vi "drive_getInputs.vi"(11 "Joysticks":T2) -> (3 "Drive":T1)   [LabVIEW 2013]
uses:
  util/joystick_vals.ctl
  <vilib>/Rock Robotics/WPI/Joystick/WPI_JoystickButtonState.ctl
  drive_inputs.ctl
panel:
  out "Angular Rate":dbl
  in  "Drive 2":T1
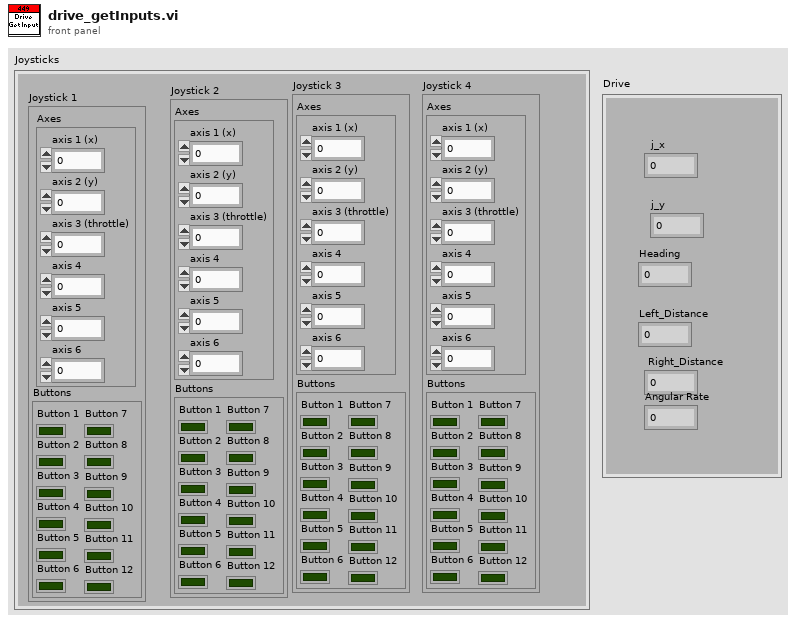
[diagram p1: front panel]
types:
  T1 = typedef "drive_inputs.ctl" = cluster{"j_x":dbl, "j_y":dbl, "Heading":dbl, "Left_Distance":dbl, " Right_Distance":dbl}
  T2 = typedef "joystick_vals.ctl" = cluster{"Joystick 1":cluster{"Axes":cluster{"axis 1 (x)":dbl, "axis 2 (y)":dbl, "axis 3 (throttle)":dbl, "axis 4":dbl, "axis 5":dbl, "axis 6":dbl}, "Buttons":T3}, "Joystick 2":cluster{"Axes":cluster{"axis 1 (x)":dbl, "axis 2 (y)":dbl, "axis 3 (throttle)":dbl, "axis 4":dbl, "axis 5":dbl, "axis 6":dbl}, "Buttons":T3}, "Joystick 3":cluster{"Axes":cluster{"axis 1 (x)":dbl, "axis 2 (y)":dbl, "axis 3 (throttle)":dbl, "axis 4":dbl, "axis 5":dbl, "axis 6":dbl}, "Buttons":T3}, "Joystick 4":cluster{"Axes":cluster{"axis 1 (x)":dbl, "axis 2 (y)":dbl, "axis 3 (throttle)":dbl, "axis 4":dbl, "axis 5":dbl, "axis 6":dbl}, "Buttons":T3}}
  T3 = typedef "WPI_JoystickButtonState.ctl" = cluster{"Button 1":bool, "Button 2":bool, "Button 3":bool, "Button 4":bool, "Button 5":bool, "Button 6":bool, "Button 7":bool, "Button 8":bool, "Button 9":bool, "Button 10":bool, "Button 11":bool, "Button 12":bool}
  T4 = cluster{"Axes":cluster{"axis 1 (x)":dbl, "axis 2 (y)":dbl, "axis 3 (throttle)":dbl, "axis 4":dbl, "axis 5":dbl, "axis 6":dbl}, "Buttons":T3}
  T5 = cluster{"axis 1 (x)":dbl, "axis 2 (y)":dbl, "axis 3 (throttle)":dbl, "axis 4":dbl, "axis 5":dbl, "axis 6":dbl}
  T6 = typedef "WPI_EncoderDevRef.ctl" = cluster{"DevStatus":errorcluster, "EncoderIndex":T7, "CounterIndex":T8, "DistancePerCount":dbl, "Decoding Type":T9}
  T7 = typedef "FPGA_EncoderIdx.ctl" = enum8{"Enc 0", "Enc 1", "Enc 2", "Enc 3", "Invalid"}
  T8 = typedef "FPGA_CounterCtrSystemIndex.ctl" = enum8{"Ctr 0", "Ctr 1", "Ctr 2", "Ctr 3", "Ctr 4", "Ctr 5", "Ctr 6", "Ctr 7", "Invalid"}
  T9 = typedef "WPI_EncoderType.ctl" = enum16{"1x", "2x", "4x"}
  T10 = typedef "WPI_GyroDevRef.ctl" = cluster{"DevStatus":errorcluster, "Analog Module":T11, "Analog Channel":T12, "Offset":dbl, "Gain (VoltsPerDegree/Second)":dbl}
  T11 = typedef "FPGA_TypedefAnalogModule.ctl" = enum16{"Analog Module 1", "Analog Module 2"}
  T12 = typedef "FPGA_AIChannel.ctl" = enum8{"AI 1", "AI 2", "AI 3", "AI 4", "AI 5", "AI 6", "AI 7", "AI 8", "Invalid"}
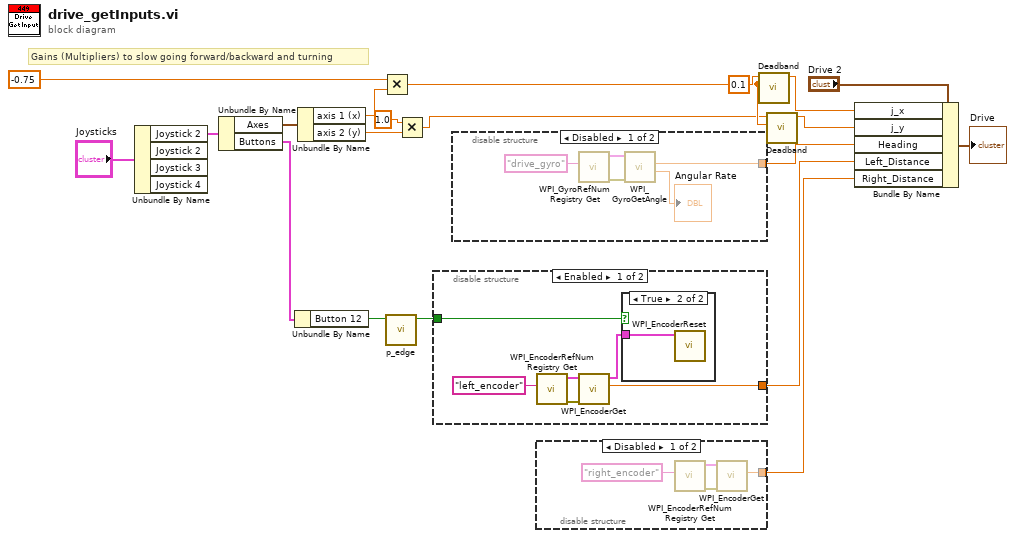
[diagram p0: block diagram]
diagram:
  w3 = 0.1 ("Deadband")
  # "Gains (Multipliers) to slow going forward/backward and turning"
  n1 = Unbundle By Name("Joysticks") -> ("Joystick 2"=w17:T4)  [unwired: 3 out]
  n2 = Unbundle By Name(w17) -> ("Axes"=w16:T5, "Buttons"=w8:T3)
  n3 = Unbundle By Name(w8) -> ("Button 12"=w7:bool)
  n4 = Unbundle By Name(w16) -> ("axis 1 (x)"=w15:dbl, "axis 2 (y)"=w14:dbl)
  n5 = Multiply(x=-0.75, y=w15) -> (x*y=w4:dbl)
  n6 = call "p_edge.vi"("In"=w7) -> ("Out"=w6:bool)  [unwired: 10 in]
  n7 = Multiply(x=1.0, y=w14) -> (x*y=w2:dbl)
  n8 = disable-structure shown="Enabled" {
    disable-tunnel: [w24 _] -> w10
    disable-tunnel: w6 -> [w21 _]
    frame Enabled {
      n9 = call <vilib>:"WPI_EncoderRefNum Registry Get.vi"("refnum name"="left_encoder") -> ("error out"=w26:errorcluster, "EncoderDevRef"=w25:T6)  [unwired: 9 in]
      n10 = call <vilib>:"WPI_EncoderGet.vi"("error in (no error)"=w26, "EncoderDevRef"=w25) -> ("Distance"=w24:dbl, "EncoderDevRef"=w22:T6)  [unwired: 4 in, 4 out]
      n11 = case shown="True" w21 {
        tunnel: w22 -> [_ w27]
        frame False {
        }
        frame True {
          n12 = call <vilib>:"WPI_EncoderReset.vi"("EncoderDevRef"=w27) -> ()  [unwired: 9 in, 2 out]
        }
      }
    }
    frame Disabled {
    }
  }
  n13 = disable-structure shown="Disabled" {
    disable-tunnel: [w30 _] -> w13
    frame Disabled {
      n14 = call <vilib>:"WPI_GyroRefNum Registry Get.vi"("refnum name"="drive_gyro") -> ("error out"=w32:errorcluster, "GyroDevRef"=w31:T10)  [unwired: 9 in]
      n15 = call <vilib>:"WPI_GyroGetAngle.vi"("error in (no error)"=w32, "GyroDevRef"=w31) -> ("Angular Rate"=→"Angular Rate":dbl, "Angle"=w30:dbl)  [unwired: 6 in, 2 out]
    }
    frame Enabled {
    }
  }
  n16 = disable-structure shown="Disabled" {
    disable-tunnel: [w34 _] -> w9
    frame Disabled {
      n17 = call <vilib>:"WPI_EncoderRefNum Registry Get.vi"("refnum name"="right_encoder") -> ("error out"=w36:errorcluster, "EncoderDevRef"=w35:T6)  [unwired: 9 in]
      n18 = call <vilib>:"WPI_EncoderGet.vi"("error in (no error)"=w36, "EncoderDevRef"=w35) -> ("Distance"=w34:dbl)  [unwired: 4 in, 5 out]
    }
    frame Enabled {
    }
  }
  n19 = call "Deadband.vi"("Deadband"=w3, "Input"=w4) -> ("Output"=w5:dbl)  [unwired: 9 in]
  n20 = call "Deadband.vi"("Deadband"=w3, "Input"=w2) -> ("Output"=w1:dbl)  [unwired: 9 in]
  n21 = Bundle By Name(cluster="Drive 2", "j_x"=w5, "j_y"=w1, "Heading"=w13, "Left_Distance"=w10, "Right_Distance"=w9) -> (→"Drive":T1)
